vi "DFD Load from File.vi"   [LabVIEW 2017, in "NI_DigFilterLicensed.lvlib"]
doc: "Retrieves a filter or a filter bank from a file. You must manually select the polymorphic instance you want to use."
uses:
  <vilib>/addons/Digital Filter Design/NI_DigFilterLicensed.lvlib
  <vilib>/addons/Digital Filter Design/NI_DigFilter_FilterBank.lvlib
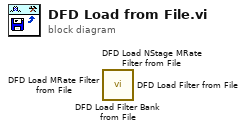
[diagram p0: block diagram]
diagram:
  n1 = call <vilib>:"DFD Load Filter Bank from File.vi"() -> ()  [unwired: 9 in, 3 out]
  n2 = call <vilib>:"DFD Load NStage MRate Filter from File.vi"() -> ()  [unwired: 9 in, 3 out]
  n3 = call <vilib>:"DFD Load MRate Filter from File.vi"() -> ()  [unwired: 9 in, 3 out]
  n4 = call <vilib>:"DFD Load Filter from File.vi"() -> ()  [unwired: 9 in, 3 out]
